vi "Manager QueryClockStatus.vi"(6 "contextId":T1, 8 "error in":errorcluster, 9 "timeout (ms)":i32=-1, 10 "Request Data":T7, 11 "gRPC ID":T1) -> (0 "error out":errorcluster, 2 "Response Data":T2, 3 "gRPC ID out":T1)   [LabVIEW 2021, in "CIF_Manager_client.lvlib"]
uses:
  CIF_Manager_client.lvlib
  <vilib>/gRPC/LabVIEW gRPC Library/Shared/grpcId.ctl
  RPC Messages/cif_manager_QueryClockStatusRequest.ctl
  RPC Messages/cif_manager_QueryClockStatusResponse.ctl
  RPC Messages/cif_manager_ClockStatusArray.ctl
  RPC Messages/cif_manager_ClockStatus.ctl
  RPC Messages/cif_manager_ClockConversion.ctl
  RPC Messages/cif_manager_TimePair.ctl
  RPC Messages/cif_manager_QueryClockStatusResponse_Flat.ctl
  RPC Messages/cif_manager_ClockStatusArray_Flat.ctl
  RPC Messages/cif_manager_ClockStatus_Flat.ctl
  RPC Messages/cif_manager_ClockConversion_Flat.ctl
  RPC Messages/cif_manager_TimePair_Flat.ctl
  14035477-4c25-4107-8ed5-d0c4ef420ce5.vi
  <vilib>/gRPC/LabVIEW gRPC Library/Shared/TranslateGrpcError.vi
  <vilib>/gRPC/LabVIEW gRPC Library/Shared/Wait On Occurrence.vi
  RPC Messages/FlatToRichcif_manager_ClockStatusArray.vi
  <vilib>/gRPC/LabVIEW gRPC Library/Shared/Is Feature Enabled.vi
  RPC Messages/FlatToRichcif_manager_ClockStatus.vi
  RPC Messages/FlatToRichcif_manager_ClockConversion.vi
  RPC Messages/FlatToRichcif_manager_TimePair.vi
  <vilib>/gRPC/LabVIEW gRPC Library/Server API/Server/Get Server DLL Path.vi
  <vilib>/Utility/error.llb/Error Cluster From Error Code.vi
  <vilib>/gRPC/LabVIEW gRPC Library/grpc-lvsupport-release.lvlib
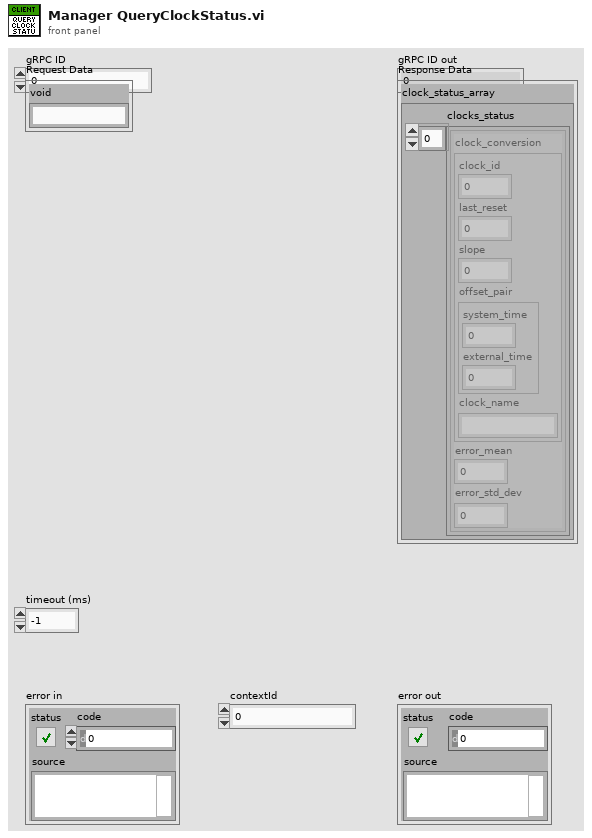
[diagram p1: front panel]
types:
  T1 = typedef "grpc-lvsupport-release.lvlib/grpcId.ctl" = u64
  T2 = typedef "CIF_Manager_client.lvlib/cif_manager_QueryClockStatusResponse.ctl" = cluster{"clock_status_array":T3}
  T3 = typedef "CIF_Manager_client.lvlib/cif_manager_ClockStatusArray.ctl" = cluster{"clocks_status":T4[]}
  T4 = typedef "CIF_Manager_client.lvlib/cif_manager_ClockStatus.ctl" = cluster{"clock_conversion":T5, "error_mean":i64, "error_std_dev":i64}
  T5 = typedef "CIF_Manager_client.lvlib/cif_manager_ClockConversion.ctl" = cluster{"clock_id":u32, "last_reset":i64, "slope":dbl, "offset_pair":T6, "clock_name":string}
  T6 = typedef "CIF_Manager_client.lvlib/cif_manager_TimePair.ctl" = cluster{"system_time":i64, "external_time":i64}
  T7 = typedef "CIF_Manager_client.lvlib/cif_manager_QueryClockStatusRequest.ctl" = cluster{"void":string}
  T8 = typedef "CIF_Manager_client.lvlib/cif_manager_QueryClockStatusResponse_Flat.ctl" = cluster{"clock_status_array":T9}
  T9 = typedef "CIF_Manager_client.lvlib/cif_manager_ClockStatusArray_Flat.ctl" = cluster{"clocks_status":T10[]}
  T10 = typedef "CIF_Manager_client.lvlib/cif_manager_ClockStatus_Flat.ctl" = cluster{"clock_conversion":T11, "error_mean":i64, "error_std_dev":i64}
  T11 = typedef "CIF_Manager_client.lvlib/cif_manager_ClockConversion_Flat.ctl" = cluster{"clock_id":u32, "last_reset":i64, "slope":dbl, "offset_pair":T12, "clock_name":string}
  T12 = typedef "CIF_Manager_client.lvlib/cif_manager_TimePair_Flat.ctl" = cluster{"system_time":i64, "external_time":i64}
  T13 = typedef "CIF_Manager_client.lvlib/cif_manager_QueryClockStatusRequest_Flat.ctl" = cluster{"void":string}
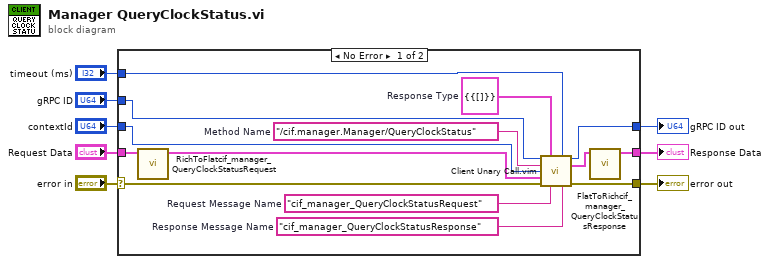
[diagram p0: block diagram]
diagram:
  n1 = case shown="No Error" "error in" {
    selector: "error in" -> [w18 w23]
    tunnel: [w17 w23] -> w7
    tunnel: "gRPC ID" -> [w16 w24]
    tunnel: [w15 w24] -> w5
    tunnel: "Request Data" -> [w12 _]
    tunnel: [w9 _] -> w3
    tunnel: "timeout (ms)" -> [w14 _]
    tunnel: "contextId" -> [w13 _]
    frame No Error {
      w19 = "cif_manager_QueryClockStatusResponse"  # Response Message Name
      w20 = "cif_manager_QueryClockStatusRequest"  # Request Message Name
      w21 = T8 {"clock_status_array"={"clocks_status"=[]}}  # Response Type
      w22 = "/cif.manager.Manager/QueryClockStatus"  # Method Name
      n2 = call "RichToFlatcif_manager_QueryClockStatusRequest.vi"("InputCluster"=w12) -> ("OutputCluster"=w11:T13)  [unwired: 10 in]
      n3 = call "Client Unary Call.vim"("ClientID in"=w16, "Response Type"=w21, "timeout (ms)"=w14, "Method Name"=w22, "contextId"=w13, "Request Data"=w11, "error in"=w18, "Request Message Name"=w20, "Response Message Name"=w19) -> ("ClientID out"=w15:u64, "Response Data"=w10:T8, "error out"=w17:errorcluster)  [unwired: 4 in]
      n4 = call "FlatToRichcif_manager_QueryClockStatusResponse.vi"("InputCluster"=w10) -> ("OutputCluster"=w9:T2)  [unwired: 10 in]
    }
    frame Error {
    }
  }
  "error out" <- w7
  "gRPC ID out" <- w5
  "Response Data" <- w3
